vi "Read.vi"(7 "Slave Address":u8, 8 "Error In":errorcluster, 10 "Count":i32, 11 "LINX I2C In":refnum<class "LINX I2C.lvclass">) -> (0 "Error Out":errorcluster, 2 "Data":u8[](array[numeric]), 3 "LINX I2C Out":refnum<class "LINX I2C.lvclass">)   [LabVIEW 2020, in "lv_i2c_linx.lvlib" / "LINX I2C.lvclass"]
uses:
  LINX I2C.lvclass
  LINX I2C.lvclass/LINX I2C.ctl
  <vilib>/MakerHub/LINX/LMH-LINX.lvlib
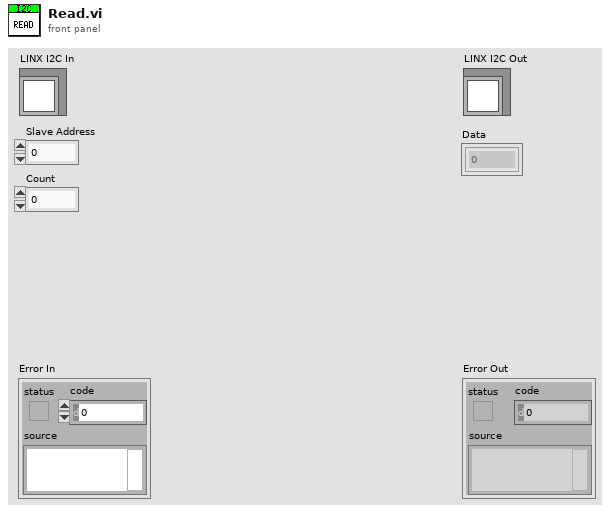
[diagram p1: front panel]
types:
  T1 = typedef "LMH-LINX.lvlib/LINX Ref.ctl" = cluster{"IO":T2, "Interface":T3, "LINX Device Config":T4}
  T2 = typedef "LMH-LINX.lvlib/Platform.ctl" = enum16{"Remote", "Local"}
  T3 = typedef "LMH-LINX.lvlib/Interface.ctl" = enum16{"Serial", "TCP"}
  T4 = typedef "LMH-LINX.lvlib/Device.lvlib/LINX Device Config.ctl" = cluster{"Interface":T3, "COM Port":refnum<visa-resource-name>, "TCP Configuration":T5, "Device Family":u8, "Device ID":u8, "Device Name":string, "TCP Ref":refnum<k5>, "Channels":T6}
  T5 = typedef "LMH-LINX.lvlib/Device.lvlib/TCP Config.ctl" = cluster{"IP Address":string, "Port":u16}
  T6 = typedef "LMH-LINX.lvlib/Channels.ctl" = cluster{"DI":u8[], "DO":u8[], "AI":u8[], "AO":u8[], "PWM":u8[], "QE":u8[], "UART":u8[], "I2C 2":u8[], "SPI":u8[], "CAN":u8[], "Servo":u8[], "AI Ref (V)":dbl, "AI Resolution (Bits)":u8, "AO Ref (V)":dbl, "AO Resolution (Bits)":u8}
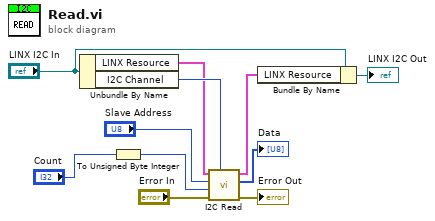
[diagram p0: block diagram]
diagram:
  n1 = Unbundle By Name("LINX I2C In") -> ("LINX Resource"=w6:T1, "I2C Channel"=w7:u8)
  n2 = To Unsigned Byte Integer(number="Count") -> (unsigned 8bit integer=w1:u8)
  n3 = call <vilib>:"I2C Read.vi"("I2C Channel"=w7, "Error In"="Error In", "Bytes To Read"=w1, "I2C Slave Address (0)"="Slave Address", "LINX Resource"=w6) -> ("Error Out"=→"Error Out":errorcluster, "Data"=→"Data":u8[], "LINX Resource"=w4:T1)  [unwired: 4 in]
  n4 = Bundle By Name(cluster="LINX I2C In", "LINX Resource"=w4) -> (→"LINX I2C Out":refnum<class "LINX I2C.lvclass">)
